vi "rgb_to_gray.vi"(11 "24-bit pixmap":u32[][](array[numeric])) -> (3 "Array":u32[][](array[numeric]))   [LabVIEW 2023]
doc: "Converts RGB picture to grayscale."
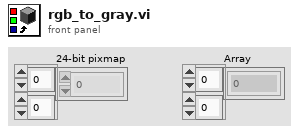
[diagram p1: front panel]
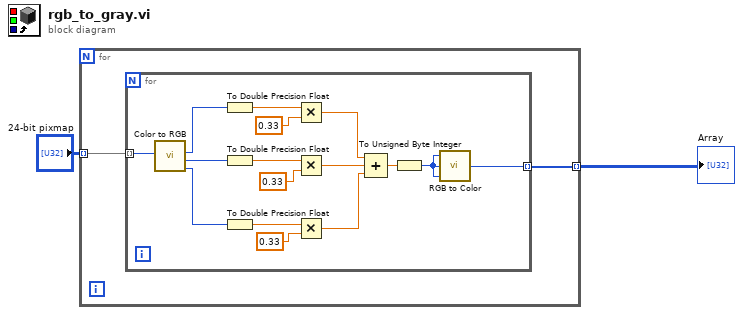
[diagram p0: block diagram]
diagram:
  n1 = for {
    tunnel: "24-bit pixmap" -> [w4] mode=indexing
    tunnel: [w3] -> w2 mode=indexing
    n2 = for {
      tunnel: w4 -> [w20] mode=indexing
      tunnel: [w5] -> w3 mode=indexing
      n3 = call <vilib>:"Color to RGB.vi"("Color"=w20) -> ("R"=w19:u8, "G"=w18:u8, "B"=w17:u8)  [unwired: 1 out]
      n4 = To Double Precision Float(number=w19) -> (double precision float=w16:dbl)
      n5 = To Double Precision Float(number=w18) -> (double precision float=w14:dbl)
      n6 = To Double Precision Float(number=w17) -> (double precision float=w12:dbl)
      n7 = Multiply(x=w16, y=0.33) -> (x*y=w10:dbl)
      n8 = Multiply(x=w14, y=0.33) -> (x*y=w9:dbl)
      n9 = Multiply(x=w12, y=0.33) -> (x*y=w8:dbl)
      n10 = Compound Arithmetic op=ADD(w10, w9, w8) -> (w7:dbl)
      n11 = To Unsigned Byte Integer(number=w7) -> (unsigned 8bit integer=w6:u8)
      n12 = call <vilib>:"RGB to Color.vi"("B"=w6, "G"=w6, "R"=w6) -> ("Color"=w5:u32)
    }
  }
  "Array" <- w2
